vi "U16ToByte.vi"(11 "数值":u16) -> (2 "高8位":u8, 3 "低8位":u8)   [LabVIEW 2018]
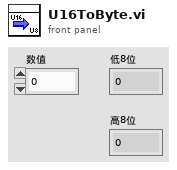
[diagram p1: front panel]
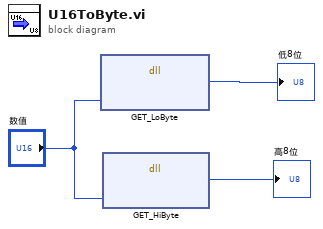
[diagram p0: block diagram]
diagram:
  n1 = dll-call lib="PTH2qabs CUsersadminDesktopzlgcan_demo_20220516_2018版本zlgcan_demo_USBCANFD_mergebinzlgcan_wrap.dll" fn="GET_LoByte"("U16(IN)"="数值") -> ("返回类型"=→"低8位":u8)  [unwired: 4 in, 2 out]
  n2 = dll-call lib="PTH2qabs CUsersadminDesktopzlgcan_demo_20220516_2018版本zlgcan_demo_USBCANFD_mergebinzlgcan_wrap.dll" fn="GET_HiByte"("U16(IN)"="数值") -> ("返回类型"=→"高8位":u8)  [unwired: 4 in, 2 out]
